vi "TEST_TRAJECTORY_SAMPLE.vi"() -> ()   [LabVIEW 2019]
uses:
  Robot Global Data.vi
  <vilib>/Rock Robotics/WPI/ThirdParty/JAS_Junk/TrajLib/Trajectory_Library.lvlib
panel:
  in  "Tab Control":T1(tab)
  in  "Read FIle\nand Plot":bool
  in  "Trajectory File Name":path=path "Sample-Robot-2-Trajectory-TrajLibrary.csv"
  out "Traj File Good":bool
  out "read file error":errorcluster
  out "Lib Rev":cluster{dbl[], dbl[]}[](graph)
  out "Custom Follow Rev":cluster{dbl[], dbl[]}[](graph)
  out "Custom Const Rev":cluster{dbl[], dbl[]}[](graph)
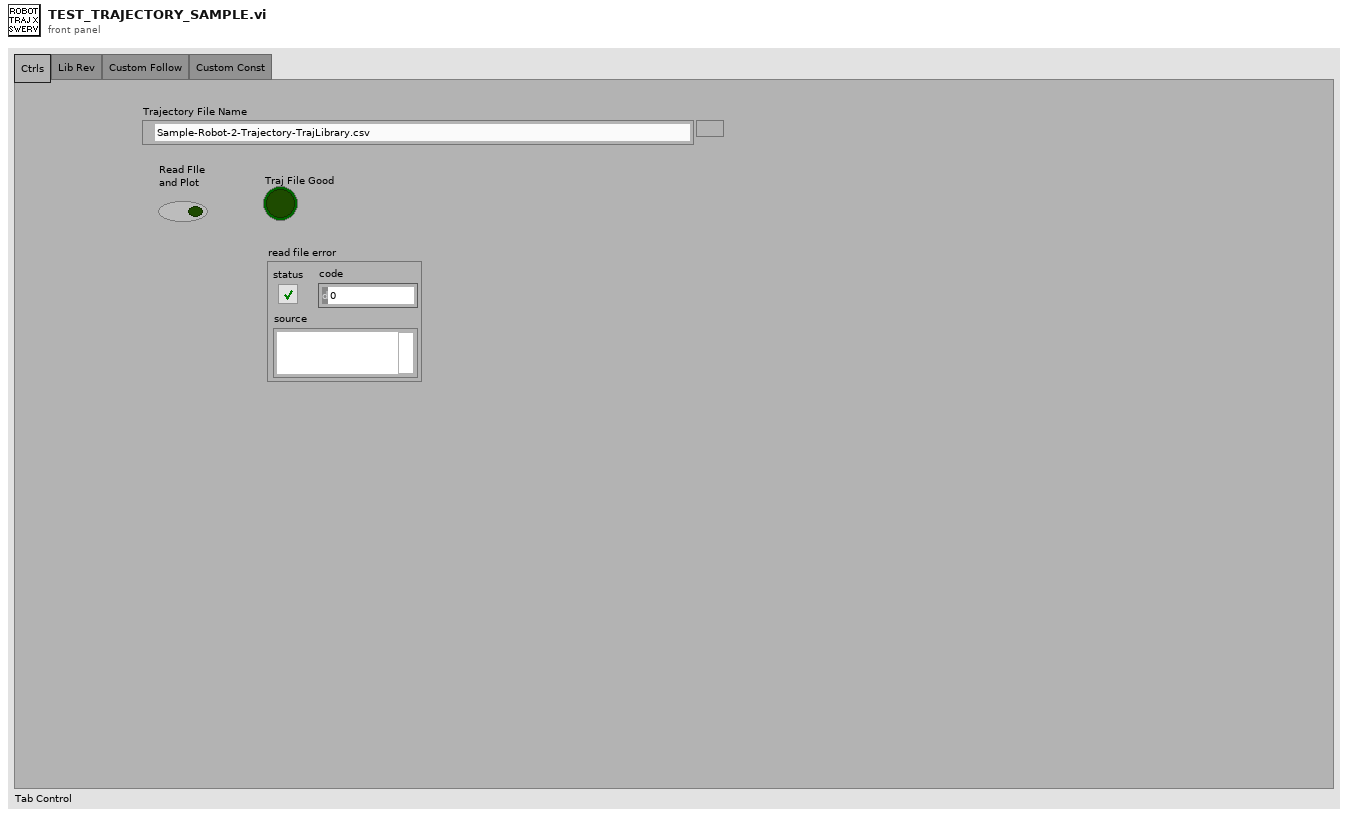
[diagram p1: front panel]
types:
  T1 = enum32{"Ctrls", "Lib Rev", "Custom Follow", "Custom Const"}
  T2 = typedef "Trajectory_Library.lvlib/TRAJECTORY.ctl" = cluster{"TotalTImeSecs":dbl, "States":T3[]}
  T3 = typedef "Trajectory_Library.lvlib/TRAJ_STATE.ctl" = cluster{"TimeSeconds":dbl, "Velocity":dbl, "Acceleration":dbl, "POSE":T4, "Curvature":dbl}
  T4 = typedef "Trajectory_Library.lvlib/POSE2D.ctl" = cluster{"TRANSLATION":T5, "ROTATION":T6}
  T5 = typedef "Trajectory_Library.lvlib/TRANSLATION2D.ctl" = cluster{"X":dbl, "Y":dbl}
  T6 = typedef "Trajectory_Library.lvlib/ROTATION2D.ctl" = cluster{"VALUE":dbl, "COS":dbl, "SIN":dbl}
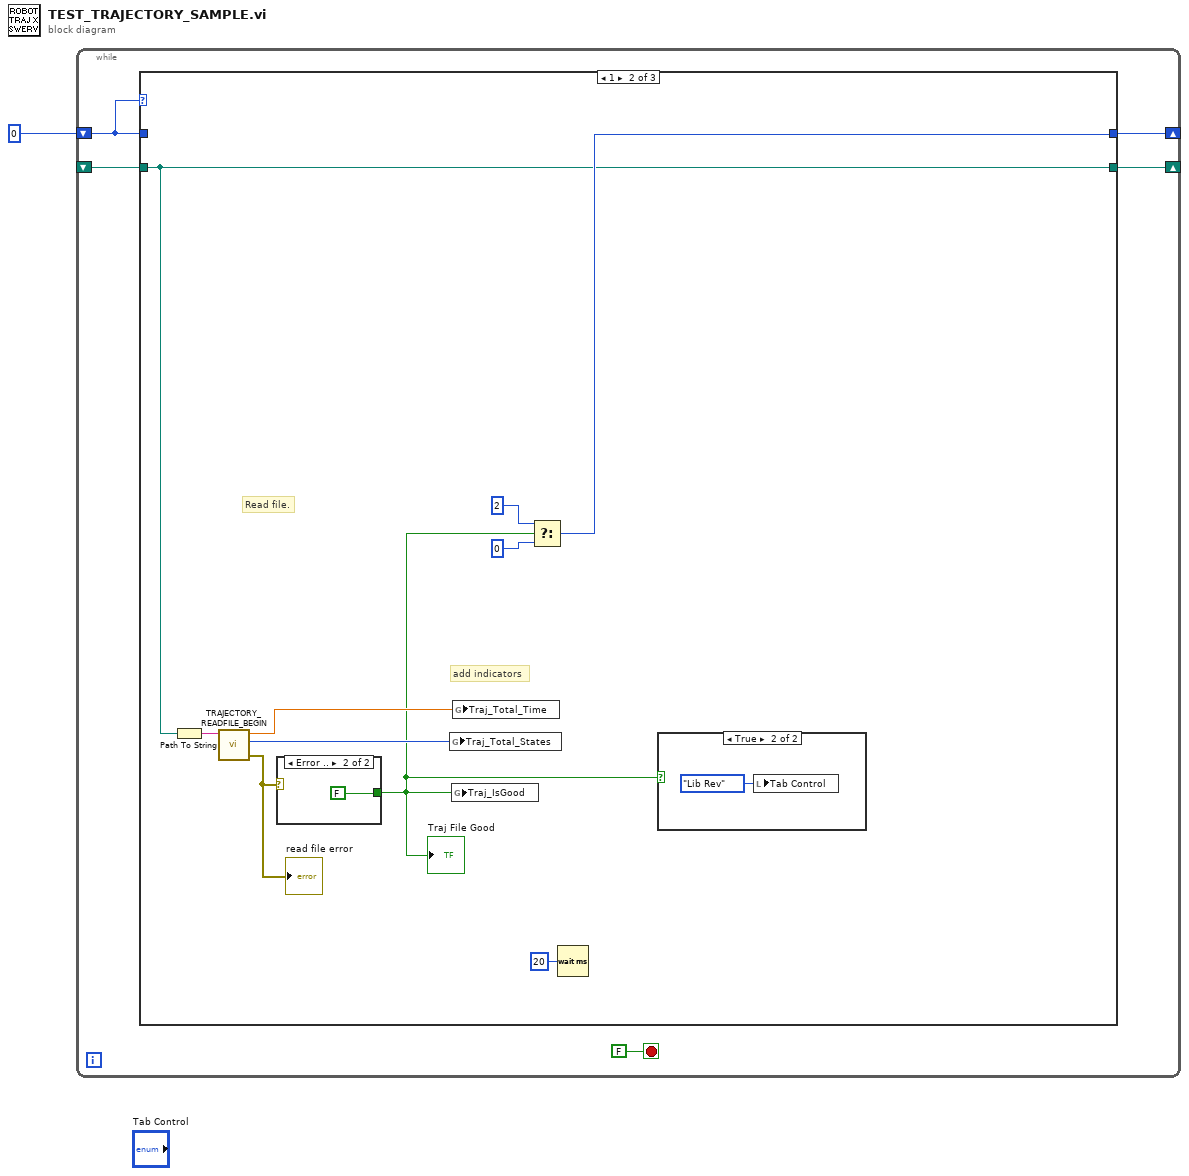
[diagram p0: block diagram]
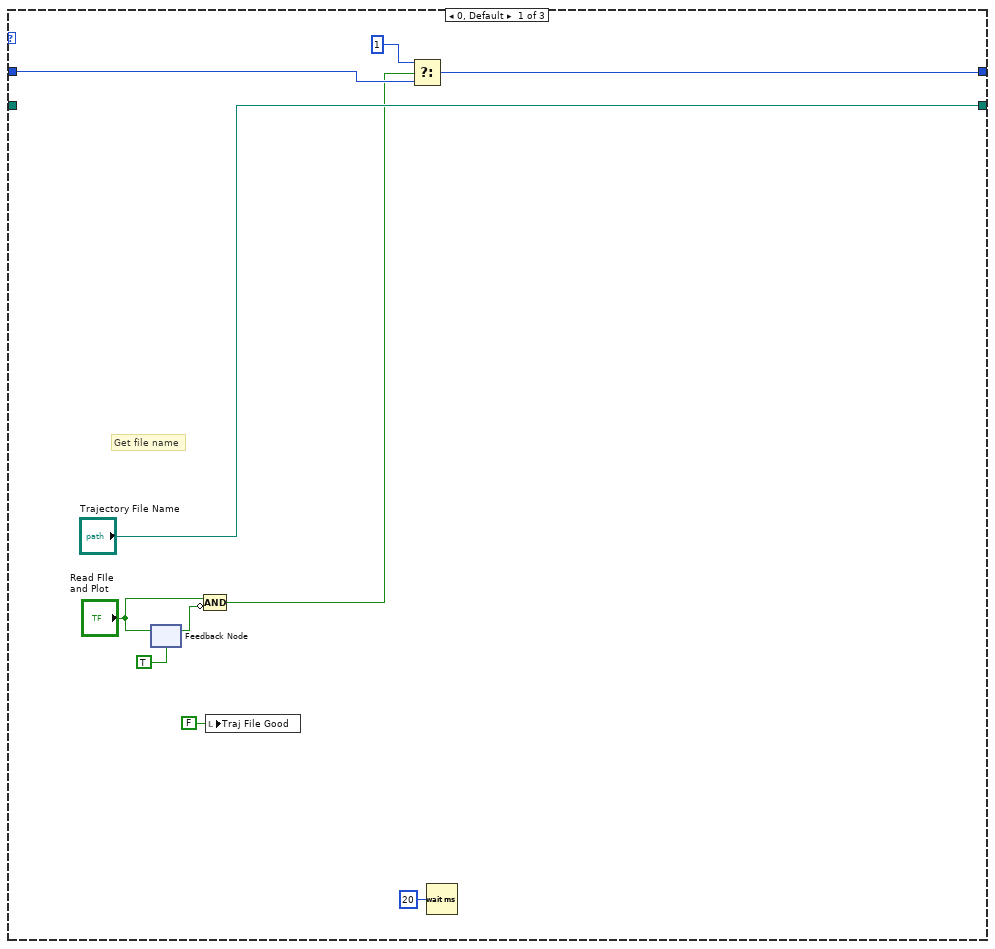
[diagram p2: hidden frame]
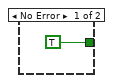
[diagram p4: hidden frame]
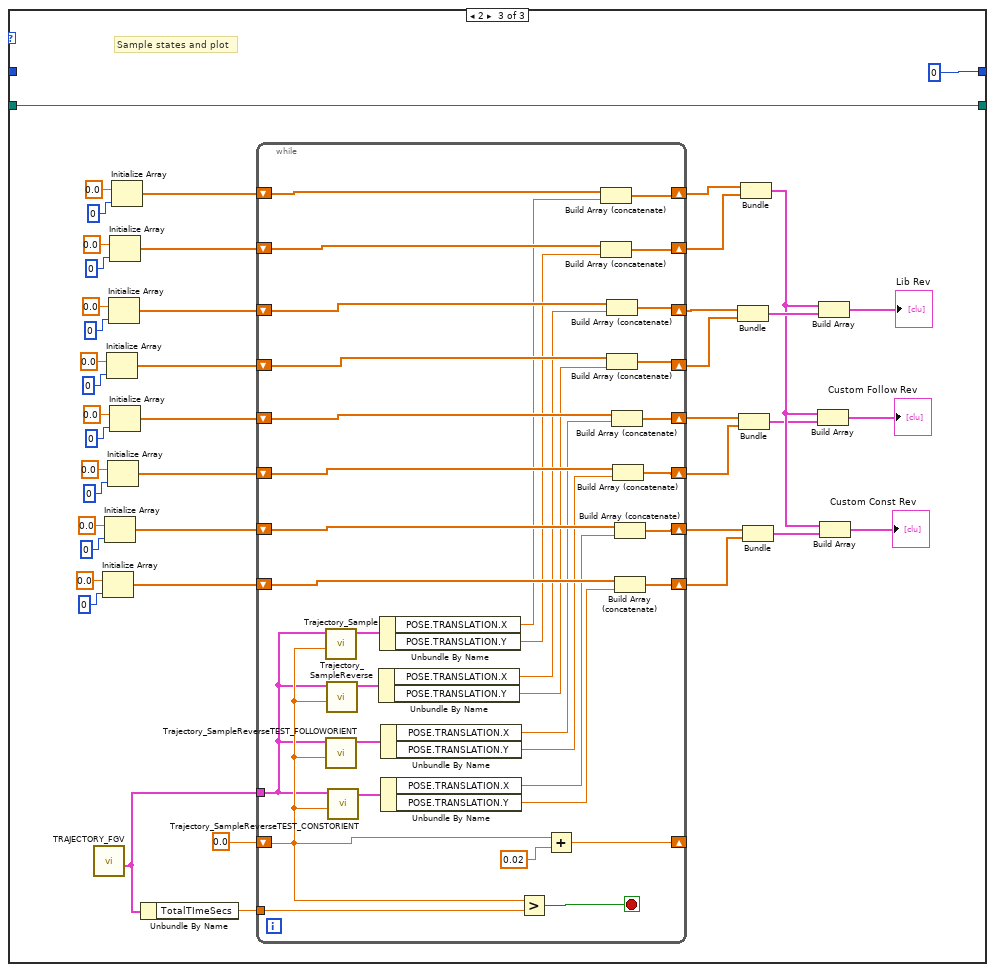
[diagram p5: hidden frame]
diagram:
  n1 = while {
    shift-right: [w5] -> _
    shift-left: 0 -> [w4]
    shift-right: [w3] -> _
    shift-left: _ -> [w2]
    stop <- FALSE stop-if-true
    n2 = case shown="1" w4 {
      tunnel: [w12 w25 0 ("f")] -> w5
      tunnel: w4 -> [w11 _ _]
      tunnel: ["Trajectory File Name" w18 w73] -> w3
      tunnel: w2 -> [_ w18 w73]
      frame 0, Default {
        # "Get file name"
        n3 = feedback #1(TRUE ("Step")) -> (w15:bool)
        n4 = feedback-in #1("Read FIle\nand Plot") -> ()
        n5 = Compound Arithmetic op=AND("Read FIle\nand Plot", invert w15) -> (w8:bool)
        n6 = local write "Traj File Good"(FALSE ("Traj File Good")) -> ()
        n7 = Select(t=1, s=w8, f=w11) -> (s? t:f=w12:i32)
        n8 = Wait (ms)(milliseconds to wait=u32 20) -> ()  [unwired: 1 out]
      }
      frame 1 {
        # "add indicators"
        # "Read file."
        n9 = Path To String(path=w18) -> (string=w19:string)
        n10 = call "TRAJECTORY_READFILE_BEGIN.vi"("Trajectory File Name"=w19) -> ("error out"=w22:errorcluster, "Trajectory Items"=w20:i32, "TotalTImeSecs"=w21:dbl)  [unwired: 8 in]
        "read file error" <- w22
        n11 = case shown="Error .." w22 {
          tunnel: [TRUE FALSE] -> w17
          frame No Error {
          }
          frame Error {
          }
        }
        "Traj File Good" <- w17
        n12 = global write "Robot Global Data.vi" "Traj_Total_States"(w20) -> ()
        n13 = global write "Robot Global Data.vi" "Traj_IsGood"(w17) -> ()
        n14 = global write "Robot Global Data.vi" "Traj_Total_Time"(w21) -> ()
        n15 = Select(t=2, s=w17, f=0) -> (s? t:f=w25:i32)
        n16 = Wait (ms)(milliseconds to wait=u32 20) -> ()  [unwired: 1 out]
        n17 = case shown="True" w17 {
          frame False {
          }
          frame True {
            n18 = local write "Tab Control"(T1."Lib Rev" ("Tab Control")) -> ()
          }
        }
      }
      frame 2 {
        # "Sample states and plot"
        n19 = call "TRAJECTORY_FGV.vi"() -> ("outTRAJECTORY"=w69:T2)  [unwired: 11 in]
        n20 = Initialize Array(0.0 ("element"), 0 ("dimension size")) -> (w45:dbl[])
        n21 = Initialize Array(0.0 ("element"), 0 ("dimension size")) -> (w46:dbl[])
        n22 = Initialize Array(0.0 ("element"), 0 ("dimension size")) -> (w49:dbl[])
        n23 = Initialize Array(0.0 ("element"), 0 ("dimension size")) -> (w47:dbl[])
        n24 = Initialize Array(0.0 ("element"), 0 ("dimension size")) -> (w50:dbl[])
        n25 = Initialize Array(0.0 ("element"), 0 ("dimension size")) -> (w51:dbl[])
        n26 = Initialize Array(0.0 ("element"), 0 ("dimension size")) -> (w48:dbl[])
        n27 = Initialize Array(0.0 ("element"), 0 ("dimension size")) -> (w52:dbl[])
        n28 = Unbundle By Name(w69) -> ("TotalTImeSecs"=w70:dbl)
        n29 = while {
          shift-right: [w107] -> _
          shift-left: 0.0 -> [w104]
          tunnel: w70 -> [w103]
          tunnel: w69 -> [w74]
          shift-right: [w97] -> w38
          shift-left: w46 -> [w84]
          shift-right: [w91] -> w44
          shift-left: w52 -> [w90]
          shift-right: [w92] -> w43
          shift-left: w51 -> [w87]
          shift-right: [w93] -> w42
          shift-left: w50 -> [w89]
          shift-right: [w94] -> w41
          shift-left: w49 -> [w88]
          shift-right: [w95] -> w40
          shift-left: w48 -> [w86]
          shift-right: [w96] -> w39
          shift-left: w47 -> [w85]
          shift-right: [w98] -> w37
          shift-left: w45 -> [w83]
          stop <- w106 stop-if-true
          n30 = call <vilib>:"Trajectory_Sample.vi"("Time"=w104, "InputTRAJECTORY"=w74) -> ("OutputTRAJ_STATE"=w102:T3)  [unwired: 9 in]
          n31 = call "Trajectory_SampleReverseTEST_FOLLOWORIENT.vi"("Time"=w104, "InputTRAJECTORY"=w74) -> ("OutputTRAJ_STATE"=w100:T3)  [unwired: 9 in]
          n32 = call <vilib>:"Trajectory_SampleReverse.vi"("Time"=w104, "InputTRAJECTORY"=w74) -> ("OutputTRAJ_STATE"=w101:T3)  [unwired: 9 in]
          n33 = call "Trajectory_SampleReverseTEST_CONSTORIENT.vi"("Time"=w104, "InputTRAJECTORY"=w74) -> ("OutputTRAJ_STATE"=w99:T3)  [unwired: 9 in]
          n34 = Unbundle By Name(w101) -> ("POSE.TRANSLATION.X"=w80:dbl, "POSE.TRANSLATION.Y"=w79:dbl)
          n35 = Unbundle By Name(w102) -> ("POSE.TRANSLATION.X"=w82:dbl, "POSE.TRANSLATION.Y"=w81:dbl)
          n36 = Unbundle By Name(w100) -> ("POSE.TRANSLATION.X"=w78:dbl, "POSE.TRANSLATION.Y"=w77:dbl)
          n37 = Unbundle By Name(w99) -> ("POSE.TRANSLATION.X"=w76:dbl, "POSE.TRANSLATION.Y"=w75:dbl)
          n38 = Greater?(x=w104, y=w103) -> (0:w106:bool)
          n39 = Add(x=w104, y=0.02) -> (x+y=w107:dbl)
          n40 = Build Array (concatenate)(w90, w82) -> (w91:dbl[])
          n41 = Build Array (concatenate)(w87, w81) -> (w92:dbl[])
          n42 = Build Array (concatenate)(w89, w80) -> (w93:dbl[])
          n43 = Build Array (concatenate)(w88, w79) -> (w94:dbl[])
          n44 = Build Array (concatenate)(w86, w78) -> (w95:dbl[])
          n45 = Build Array (concatenate)(w85, w77) -> (w96:dbl[])
          n46 = Build Array (concatenate)(w84, w76) -> (w97:dbl[])
          n47 = Build Array (concatenate)(w83, w75) -> (w98:dbl[])
        }
        n48 = Bundle(w42, w41) -> (w36:cluster{dbl[], dbl[]})  [unwired: 1 in]
        n49 = Bundle(w40, w39) -> (w33:cluster{dbl[], dbl[]})  [unwired: 1 in]
        n50 = Bundle(w44, w43) -> (w34:cluster{dbl[], dbl[]})  [unwired: 1 in]
        n51 = Bundle(w38, w37) -> (w32:cluster{dbl[], dbl[]})  [unwired: 1 in]
        n52 = Build Array(w34, w33) -> (→"Custom Follow Rev":cluster{dbl[], dbl[]}[])
        n53 = Build Array(w34, w36) -> (→"Lib Rev":cluster{dbl[], dbl[]}[])
        n54 = Build Array(w34, w32) -> (→"Custom Const Rev":cluster{dbl[], dbl[]}[])
      }
    }
  }
